vi "DeppEnableEx.vi"(8 "Error In":errorcluster, 10 "Port":i32, 11 "Device Handle":u32) -> (0 "Error Out":errorcluster, 3 "Device Handle":u32)   [LabVIEW 2011, in "LVH-Adept.lvlib" / "DEPP.lvlib"]
uses:
  DEPP.lvlib
  Private/Type Defs/Error.ctl
  Resources/depp.dll
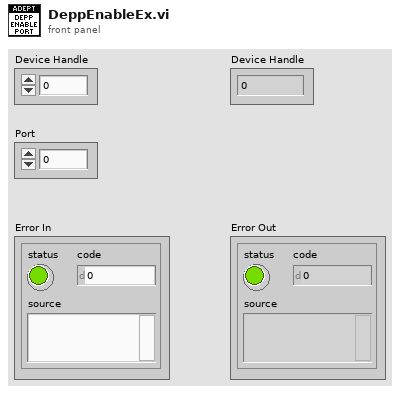
[diagram p1: front panel]
types:
  T1 = typedef "LVH-Adept.lvlib/DEPP.lvlib/Error.ctl" = enum16{"Unknown", "Enable", "Enable Port", "Get Register", "Get Register Repeat", "Get Register Set", "Put Register", "Put Register Repeat", "Put Register Set", "Disable", "Set Pair Size"}
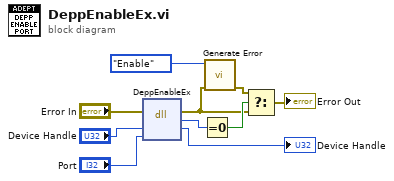
[diagram p0: block diagram]
diagram:
  n1 = dll-call lib="C:/github/labviewhacker/LVH-Adept/LabVIEW/vi.lib/LabVIEW Hacker/Adept/Private/Resources/depp.dll" fn="DeppEnableEx"(error in="Error In", "hif"="Device Handle", "prtReq"="Port") -> (error out=w2:errorcluster, "Success"=w9:u32, "hif"=→"Device Handle":u32)  [unwired: 3 in, 1 out]
  n2 = Equal To 0?(x=w9) -> (x = 0?=w8:bool)
  n3 = call "Generate Error.vi"("Error In"=w2, "DEPP Error"=Error."Enable") -> ("Error Out"=w3:errorcluster)  [unwired: 9 in]
  n4 = Select(t=w3, s=w8, f=w2) -> (s? t:f=→"Error Out":errorcluster)
